vi "Destroy Rendezvous.vi"(4 "error in (no error)":errorcluster, 7 "rendezvous":T1) -> (0 "error out":errorcluster, 3 "rendezvous name":string)   [LabVIEW 2010]
doc: "Destroys the specified rendezvous."
uses:
  Rendezvous Name & Ref DB Action.ctl
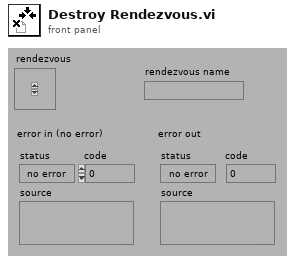
[diagram p1: front panel]
types:
  T1 = typedef "Rendezvous RefNum" = refnum<k1>
  T2 = typedef "Rendezvous Name & Ref DB Action.ctl" = enum16{"Lookup", "Insert", "Remove"}
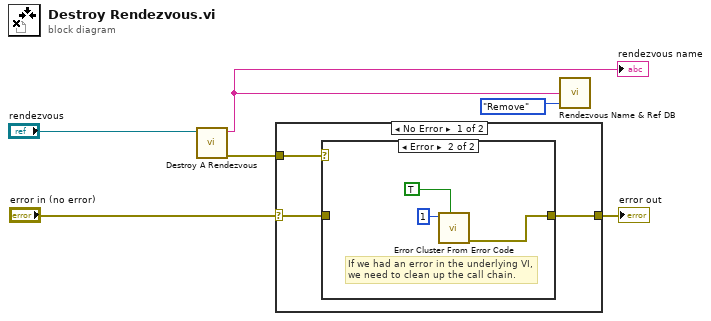
[diagram p0: block diagram]
diagram:
  n1 = call "Destroy A Rendezvous.vi"("rendezvous"="rendezvous") -> ("error out"=w2:errorcluster, "rendezvous name"=w4:string)  [unwired: 1 in, 4 out]
  "rendezvous name" <- w4
  n2 = case shown="No Error" "error in (no error)" {
    selector: "error in (no error)" -> [w7 w14]
    tunnel: [w9 w14] -> w3
    tunnel: w2 -> [w8 _]
    frame No Error {
      n3 = case shown="Error" w8 {
        tunnel: [w10 w13] -> w9
        tunnel: w7 -> [w10 _]
        frame No Error {
        }
        frame Error {
          # "If we had an error in the underlying VI,\nwe need to clean up the call chain."
          n4 = call "Error Cluster From Error Code.vi"("show call chain? (False)"=TRUE, "error code (0)"=1) -> ("error out"=w13:errorcluster)  [unwired: 1 in, 6 out]
        }
      }
    }
    frame Error {
    }
  }
  "error out" <- w3
  n5 = call "Rendezvous Name & Ref DB.vi"("Action"=Rendezvous_Name_&_Ref_DB_Action."Remove" ("Rendezvous Name & Ref DB Action"), "Rendezvous Name"=w4) -> ()  [unwired: 1 in, 1 out]
